vi "Byte Buffer.Write (String).vi"(8 "error in (no error)":errorcluster, 9 "string":string, 10 "buffer offset":u64, 11 "Byte Buffer in":refnum<class "Byte Buffer.lvclass">) -> (0 "error out":errorcluster, 2 "new buffer offset":u64, 3 "Byte Buffer out":refnum<class "Byte Buffer.lvclass">)   [LabVIEW 2016, in "VeriStand Data.lvlib" / "Byte Buffer.lvclass"]
doc: "Reads <B>count</B> elements of data from the provided <B>Byte Buffer</B> at location <B>buffer offset</B> in the format of the data type specified."
uses:
  Byte Buffer.lvclass
  Byte Buffer.lvclass/Byte Buffer.ctl
  Memory Management/Memory Management.MoveByteBlock.Read (String).vi
  Memory Management/Memory Management.Handle Return.vi
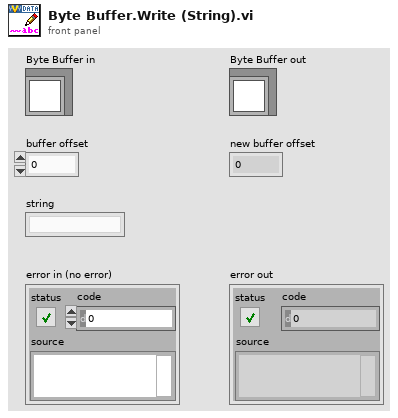
[diagram p1: front panel]
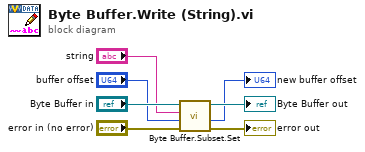
[diagram p0: block diagram]
diagram:
  n1 = call "Byte Buffer.Subset.Set.vi"("error in (no error)"="error in (no error)", "offset (0)"="buffer offset", "string in"="string", "Byte Buffer in"="Byte Buffer in") -> ("error out"=→"error out":errorcluster, "new buffer offset"=→"new buffer offset":u64, "Byte Buffer out"=→"Byte Buffer out":refnum<class "Byte Buffer.lvclass">)  [unwired: 4 in, 1 out]
